vi "Measure current noise K6430.vi"() -> ()   [LabVIEW 2014]
uses:
  <vilib>/Analysis/baseanly.llb/Mean (DBL).vi
  Environmental Chamber LabVIEW and Instruments/Drivers and Software/keithley_6430/Keithley 6430/Public/Data/Read (Single Point).vi
  <vilib>/Utility/file.llb/Write To Spreadsheet File (string).vi
  Environmental Chamber LabVIEW and Instruments/Drivers and Software/keithley_6430/Keithley 6430/Keithley 6430.lvlib
  <vilib>/Analysis/NI_AALBase.lvlib
panel:
  in  "OK Button":bool
  out "Waveform Chart":dbl(graph)
  in  "voltage settings":T1={"bias (V)"=0.001, "integration cycles"=2.0} {"integration cycles" min=0.0 format="%#_13g"}
  out "File path":path
  in  "STOP":bool
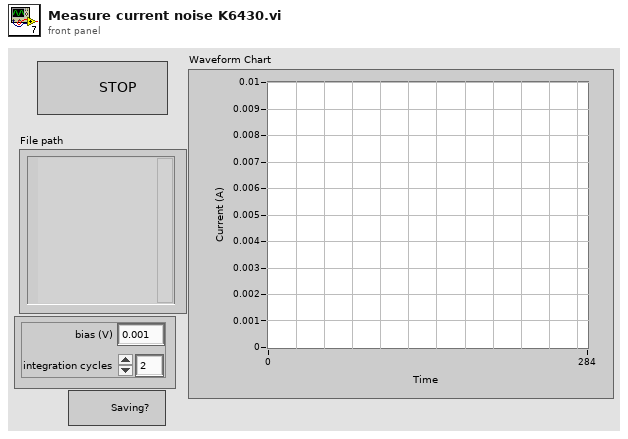
[diagram p1: front panel]
types:
  T1 = cluster{"bias (V)":dbl, "integration cycles":dbl}
  T2 = enum16{"open", "open or create", "create or replace", "create", "open (read only)"}
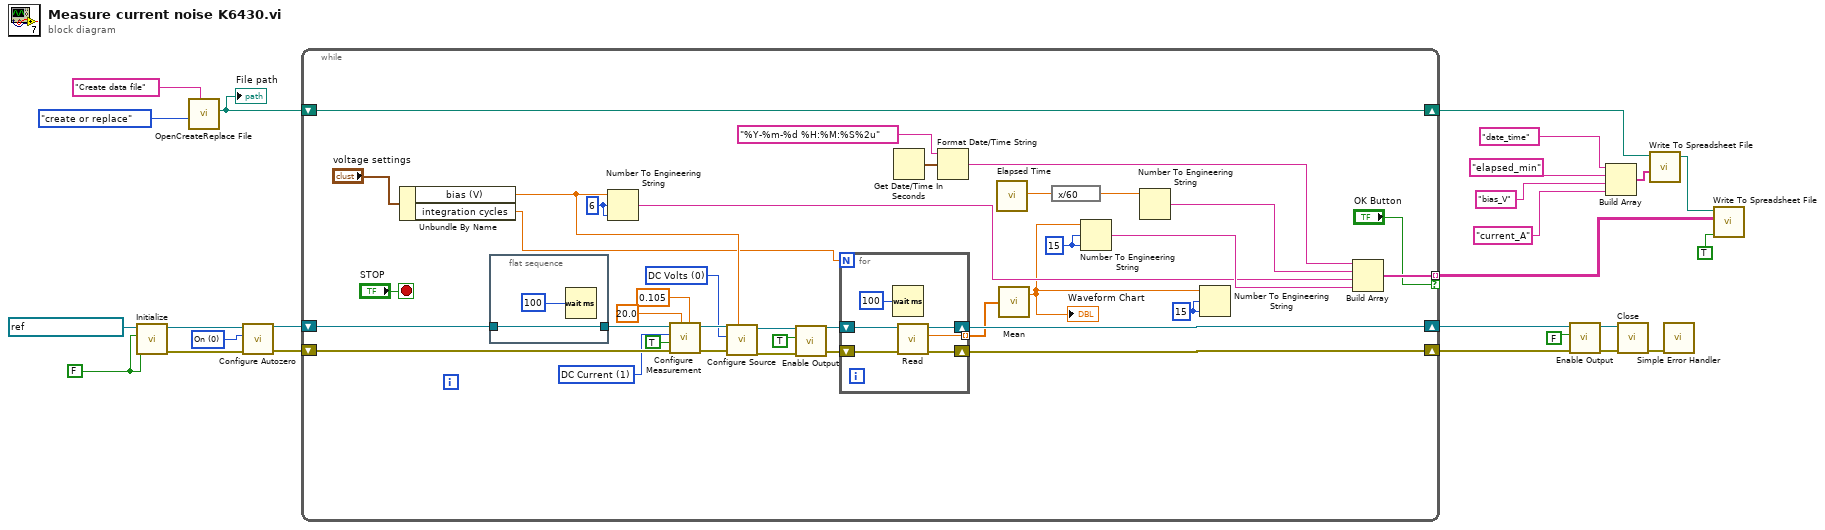
[diagram p0: block diagram]
diagram:
  w1 = FALSE ("Reset (True)")
  w19 = u16 0 items=["On", "Off", "Once"] ("Autozero  (0: On)")
  n1 = call "Initialize.vi"("Reset (True)"=w1, "ID Query (True)"=w1, "VISA resource name"=refnum<visa-resource-name> "GPIB2::19::INSTR") -> ("error out"=w18:errorcluster, "VISA resource name out"=w17:refnum<visa-resource-name>)  [unwired: 2 in, 5 out]
  n2 = call "OpenCreateReplace File.vi"("prompt"="Create data file", "function (open:0)"=T2."create or replace") -> ("new file path"=w23:path)  [unwired: 6 in, 3 out]
  "File path" <- w23
  n3 = call "Configure Autozero.vi"("error in (no error)"=w18, "Autozero  (0: On)"=w19, "VISA resource name"=w17) -> ("error out"=w9:errorcluster, "VISA resource name out"=w10:refnum<visa-resource-name>)  [unwired: 7 in]
  n4 = while {
    shift-right: [w45] -> w11
    shift-left: w9 -> [w56]
    shift-right: [w46] -> w12
    shift-left: w10 -> [w59]
    shift-right: [w62] -> w21
    shift-left: w23 -> [w62]
    tunnel: [w38] -> w3 mode=indexing if="OK Button"
    stop <- "STOP" stop-if-true
    w28 = i16 6 ("width (-)")
    w49 = u16 0 items=["DC Volts", "DC Current"] ("Source Function (0: DC Volts)")
    w50 = i16 15 ("precision (6)")
    w51 = i16 15 ("precision (6)")
    w54 = u16 1 items=["DC Volts", "DC Current"] ("Measure Function (1: DC Current)")
    n5 = Unbundle By Name("voltage settings") -> ("bias (V)"=w32:dbl, "integration cycles"=w31:dbl)
    n6 = flat-sequence {
      tunnel: w59 -> [w70]
      tunnel: [w70] -> w58
      frame #0 {
        n7 = Wait (ms)(milliseconds to wait=u32 100 ("value")) -> ()  [unwired: 1 out]
      }
    }
    n8 = Number To Engineering String(2:w28, 3:w28, 4:w32) -> (0:w39:string)  [unwired: 1 in]
    n9 = call "Configure Measurement.vi"("Current Compliance [A]"=0.105, "Voltage Compliance [V]"=20.0 ("Current Compliance [A]"), "error in (no error)"=w56, "Auto Range (T:Enable)"=TRUE, "Measure Function (1: DC Current)"=w54, "VISA resource name"=w58) -> ("error out"=w55:errorcluster, "VISA resource name out"=w57:refnum<visa-resource-name>)  [unwired: 4 in]
    n10 = call "Configure Source.vi"("V-Source Level [V]"=w32, "error in (no error)"=w55, "Source Function (0: DC Volts)"=w49, "VISA resource name"=w57) -> ("error out"=w33:errorcluster, "VISA resource name out"=w35:refnum<visa-resource-name>)  [unwired: 6 in]
    n11 = call "Enable Output.vi"("error in (no error)"=w33, "Enable Output (F:Off)"=TRUE ("Output (F:Off)"), "VISA resource name"=w35) -> ("error out"=w48:errorcluster, "VISA resource name out"=w34:refnum<visa-resource-name>)  [unwired: 7 out]
    n12 = for {
      N: w31 -> [_]
      tunnel: [w67] -> w30 mode=indexing
      shift-right: [w65] -> w45
      shift-left: w48 -> [w68]
      shift-right: [w66] -> w46
      shift-left: w34 -> [w64]
      n13 = Wait (ms)(milliseconds to wait=100 ("x")) -> ()  [unwired: 1 out]
      n14 = call-poly "Read.vi"("error in (no error)"=w68, "VISA resource name"=w64) -> ("error out"=w65:errorcluster, "Measurement"=w67:dbl, "VISA resource name out"=w66:refnum<visa-resource-name>)  [unwired: 7 in]
    }
    n15 = Get Date/Time In Seconds() -> (seconds since 1Jan1904=w61:timestamp)
    n16 = Format Date/Time String(time format string (%c)="%Y-%m-%d %H:%M:%S%2u", seconds (now)=w61) -> (date/time string=w44:string)  [unwired: 1 in]
    n17 = call "Elapsed Time"() -> ("Elapsed Time (s)"=w43:dbl)  [unwired: 12 in, 7 out]
    n18 = call-poly <vilib>:"Mean.vi"("X"=w30) -> ("mean"=w29:dbl)  [unwired: 1 out]
    "Waveform Chart" <- w29
    n19 = expression code="x/60"(w43) -> (w42:dbl)
    n20 = Number To Engineering String(2:w50, 3:w50, 4:w29) -> (0:w40:string)  [unwired: 1 in]
    n21 = Number To Engineering String(4:w42) -> (0:w41:string)  [unwired: 3 in]
    n22 = Number To Engineering String(2:w51, 3:w51, 4:w29) -> ()  [unwired: 1 in, 1 out]
    n23 = Build Array(w44, w41, w39, w40) -> (w38:string[])
  }
  n24 = call "Enable Output.vi"("error in (no error)"=w11, "Enable Output (F:Off)"=FALSE ("Output (F:Off)"), "VISA resource name"=w12) -> ("error out"=w13:errorcluster, "VISA resource name out"=w14:refnum<visa-resource-name>)  [unwired: 7 out]
  n25 = Build Array("date_time", "elapsed_min", "bias_V", "current_A") -> (w20:string[])
  n26 = call "Close.vi"("error in (no error)"=w13, "VISA resource name"=w14) -> ("error out"=w2:errorcluster)  [unwired: 9 out]
  n27 = call-poly <vilib>:"Write To Spreadsheet File.vi"("1D data"=w20, "file path (dialog if empty)"=w21) -> ("new file path (Not A Path if cancelled)"=w5:path)  [unwired: 6 in]
  n28 = call <vilib>:"Simple Error Handler.vi"("error in (no error)"=w2) -> ()  [unwired: 4 in, 5 out]
  n29 = call-poly <vilib>:"Write To Spreadsheet File.vi"("append to file? (new file:F)"=TRUE ("transpose? (no:F)"), "2D data"=w3, "file path (dialog if empty)"=w5) -> ()  [unwired: 5 in, 1 out]
